vi "ProdaNG.File.Read.vi"(6 "Config":T1={"ShowUnreleased"=FALSE, "Param1"="", "ParamStartIdx"=0, "Slots"=1} {"Slots" min=1 max=2; "ParamStartIdx" min=0 max=1}, 8 "error in (no error)":errorcluster, 9 "units":T2[](array[typedef]), 10 "SeqFile Path":path, 11 "SlotNo":i32) -> (0 "error out":errorcluster, 1 "#Slots":i32, 2 "Seq":T3)   [LabVIEW 2016]
uses:
  ProdaNG.File.Sequence.ctl
  ProdaNG.Tree.Fglb.Value.ctl
  ProdaNG.File.Step.ctl
  Controls/ProdaNG.UnitSimple.ctl
  ProdaNG.Configurator.Config.ctl
  <vilib>/Utility/config.llb/Read Key (String).vi
  <vilib>/Utility/config.llb/NI_LVConfig.lvlib
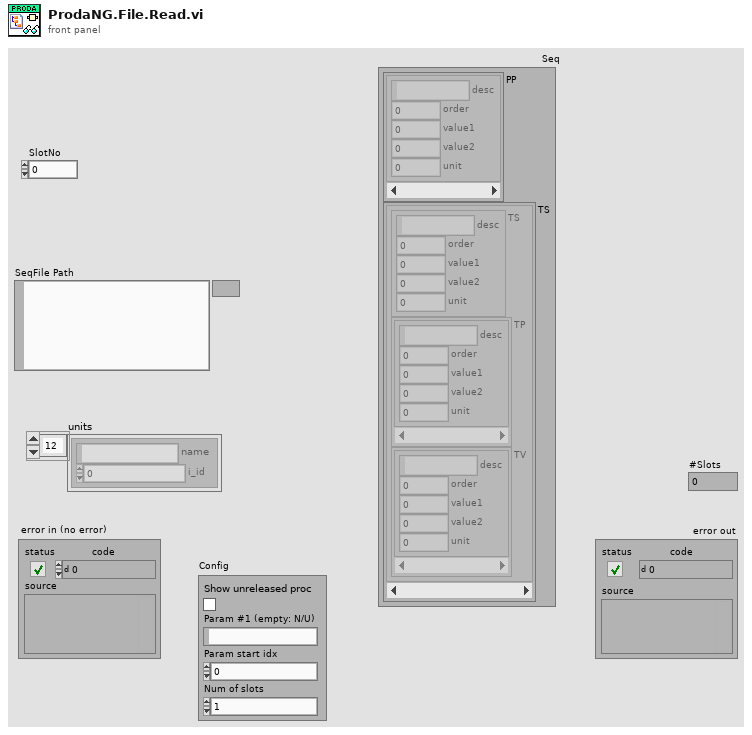
[diagram p1: front panel]
types:
  T1 = typedef "ProdaNG.Configurator.Config.ctl" = cluster{"ShowUnreleased":bool, "Param1":string, "ParamStartIdx":i32, "Slots":i32}
  T2 = typedef "ProdaNG.UnitSimple.ctl" = cluster{"name":string, "i_id":i32}
  T3 = typedef "ProdaNG.File.Sequence.ctl" = cluster{"PP":T4[], "TS":T5[]}
  T4 = typedef "ProdaNG.Tree.Fglb.Value.ctl" = cluster{"desc":string, "order":i32, "value1":dbl, "value2":dbl, "unit":i32}
  T5 = typedef "ProdaNG.File.Step.ctl" = cluster{"TS":T4, "TP":T4[], "TV":T4[]}
  T6 = typedef "NI_LVConfig.lvlib/Config Data RefNum.ctl" = refnum<k1>
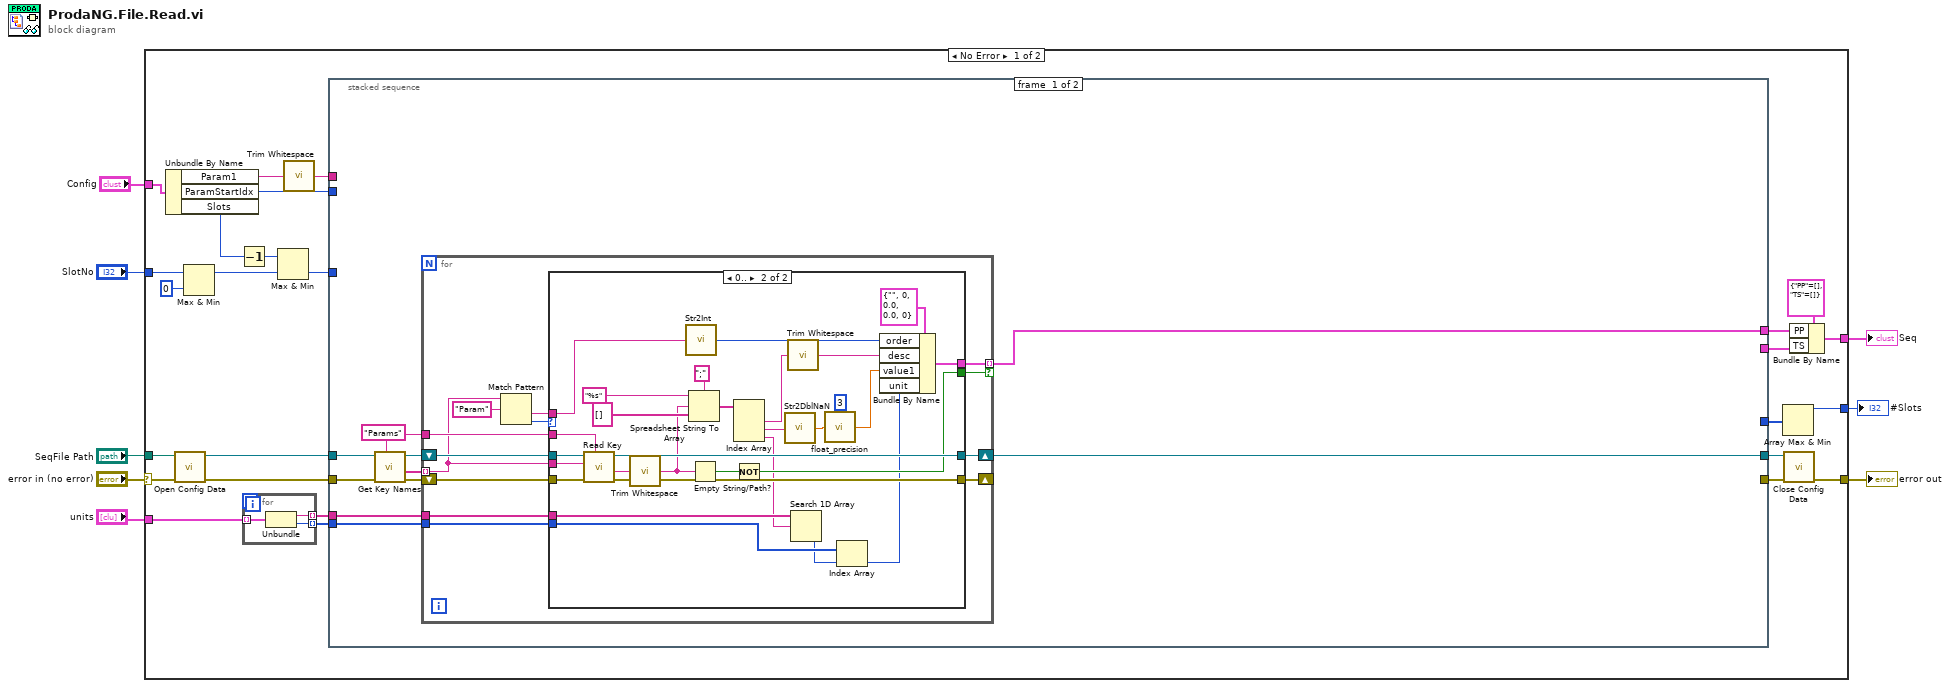
[diagram p0: block diagram]
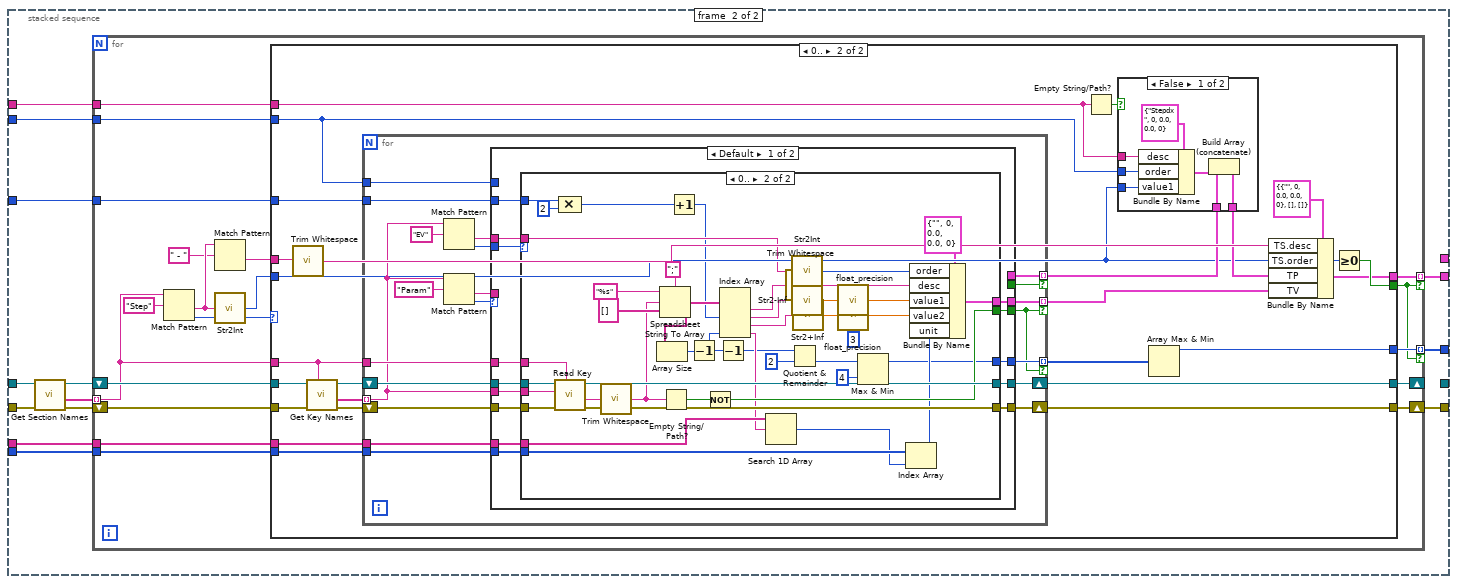
[diagram p3: hidden frame]
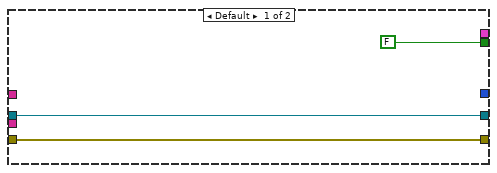
[diagram p6: hidden frame]
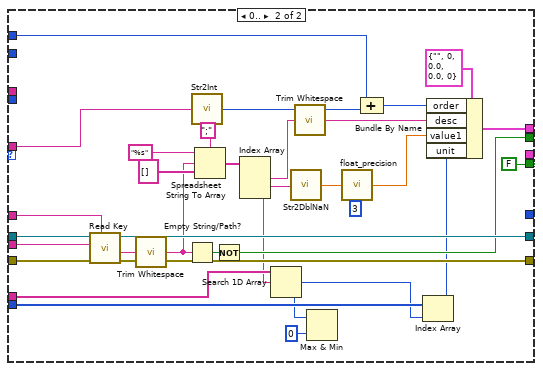
[diagram p7: hidden frame]
diagram:
  n1 = case shown="No Error" "error in (no error)" {
    selector: "error in (no error)" -> [w34 w273]
    tunnel: [w33 w273] -> w7
    tunnel: [w20 _] -> w6
    tunnel: "SeqFile Path" -> [w32 _]
    tunnel: "units" -> [w29 _]
    tunnel: "SlotNo" -> [w26 _]
    tunnel: [w18 _] -> w2
    tunnel: "Config" -> [w15 _]
    frame No Error {
      n2 = Unbundle By Name(w15) -> ("Param1"=w16:string, "ParamStartIdx"=w13:i32, "Slots"=w12:i32)
      n3 = call <vilib>:"Open Config Data.vi"("error in (no error)"=w34, "configuration file path"=w32) -> ("error out"=w31:errorcluster, "refnum"=w30:T6)  [unwired: 7 in, 1 out]
      n4 = Max & Min(x=w26, y=0) -> (max(x,y)=w10:i32)  [unwired: 1 out]
      n5 = Decrement(x=w12) -> (x-1=w11:i32)
      n6 = for {
        tunnel: [w272] -> w28 mode=indexing
        tunnel: [w271] -> w27 mode=indexing
        tunnel: w29 -> [w270] mode=indexing
        n7 = Unbundle(w270) -> ("name"=w272:string, "i_id"=w271:i32)
      }
      n8 = Max & Min(x=w11, y=w10) -> (min(x,y)=w9:i32)  [unwired: 1 out]
      n9 = call <vilib>:"Trim Whitespace.vi"("string"=w16) -> ("trimmed string"=w14:string)  [unwired: 1 in]
      n10 = stacked-sequence {
        tunnel: w31 -> [w40 w99]
        tunnel: w30 -> [w39 w98]
        tunnel: w28 -> [w38 w96]
        tunnel: w27 -> [w37 w95]
        tunnel: w9 -> [_ w94]
        tunnel: [_ w93] -> w25
        tunnel: [w36 _] -> w24
        tunnel: [_ w92] -> w22
        tunnel: [w35 _] -> w21
        tunnel: [_ w91] -> w19
        tunnel: w14 -> [_ w90]
        tunnel: w13 -> [_ w89]
        frame #0 {
          w41 = "Params" ("regular expression")
          n11 = call <vilib>:"Get Key Names.vi"("section"=w41, "error in (no error)"=w40, "refnum"=w39) -> ("error out"=w42:errorcluster, "key names"=w44:string[], "refnum out"=w43:T6)  [unwired: 5 in, 1 out]
          n12 = for {
            tunnel: w44 -> [w47] mode=indexing
            shift-right: [w50] -> w36
            shift-left: w43 -> [w54]
            shift-right: [w49] -> _
            shift-left: w42 -> [w55]
            tunnel: w41 -> [w53]
            tunnel: [w51] -> w35 mode=indexing if=w48
            tunnel: w38 -> [w46]
            tunnel: w37 -> [w45]
            n13 = Match Pattern(string=w47, regular expression="Param") -> (after substring=w52:string, offset past match=w56:i32)  [unwired: 1 in, 2 out]
            n14 = case shown="0.." w56 {
              tunnel: w55 -> [w58 w88]
              tunnel: w54 -> [w59 w87]
              tunnel: w53 -> [_ w86]
              tunnel: w47 -> [_ w85]
              tunnel: w52 -> [_ w79]
              tunnel: [_ w76] -> w51
              tunnel: [w59 w75] -> w50
              tunnel: [w58 w74] -> w49
              tunnel: [_ w71] -> w48
              tunnel: w46 -> [_ w69]
              tunnel: w45 -> [_ w67]
              frame Default {
              }
              frame 0.. {
                n15 = call-poly <vilib>:"Read Key.vi"("section"=w86, "error in (no error)"=w88, "key"=w85, "refnum"=w87) -> ("error out"=w74:errorcluster, "value"=w84:string, "refnum out"=w75:T6)  [unwired: 4 in, 1 out]
                n16 = call <vilib>:"Trim Whitespace.vi"("string"=w84) -> ("trimmed string"=w73:string)  [unwired: 1 in]
                n17 = call "Str2Int.vi"("string"=w79) -> ("Numeric"=w60:i32)
                n18 = Spreadsheet String To Array(delimiter (Tab)=";", format string="%s", spreadsheet string=w73, array type (2D Dbl)=string[] []) -> (array=w80:string[])
                n19 = Empty String/Path?(string/path=w73) -> (empty?=w72:bool)
                n20 = Index Array(array=w80) -> (element #1=w78:string, element #2=w77:string, element #3=w68:string)  [unwired: 3 in]
                n21 = Not(x=w72) -> (.not. x?=w71:bool)
                n22 = call "Str2DblNaN.vi"("string"=w77) -> ("Numeric"=w64:dbl)
                n23 = call <vilib>:"Trim Whitespace.vi"("string"=w78) -> ("trimmed string"=w65:string)  [unwired: 1 in]
                n24 = Search 1D Array(1D array=w69, element=w68) -> (index of element=w66:i32)  [unwired: 1 in]
                n25 = call "float_precision.vi"("input"=w64, "precision"=3) -> ("output"=w63:dbl)
                n26 = Index Array(array=w67, index=w66) -> (element=w61:i32)
                n27 = Bundle By Name(cluster=T4 {"desc"="", "order"=0, "value1"=0.0, "value2"=0.0, "unit"=0} ("Element values"), "order"=w60, "desc"=w65, "value1"=w63, "unit"=w61) -> (w76:T4)
              }
            }
          }
        }
        frame #1 {
          n28 = call <vilib>:"Get Section Names.vi"("error in (no error)"=w99, "refnum"=w98) -> ("error out"=w100:errorcluster, "section names"=w101:string[], "refnum out"=w97:T6)  [unwired: 7 in]
          n29 = for {
            tunnel: w101 -> [w114] mode=indexing
            shift-right: [w117] -> w93
            shift-left: w100 -> [w118]
            shift-right: [w115] -> _
            shift-left: w97 -> [w116]
            tunnel: [w113] -> w92 mode=indexing if=w104
            tunnel: w96 -> [w108]
            tunnel: w95 -> [w107]
            tunnel: w94 -> [w106]
            tunnel: [w105] -> w91 mode=indexing if=w104
            tunnel: w90 -> [w103]
            tunnel: w89 -> [w102]
            n30 = Match Pattern(string=w114, regular expression="Step") -> (after substring=w111:string, offset past match=w119:i32)  [unwired: 1 in, 2 out]
            n31 = Match Pattern(string=w111, regular expression=" - ") -> (after substring=w109:string)  [unwired: 1 in, 3 out]
            n32 = call "Str2Int.vi"("string"=w111) -> ("Numeric"=w112:i32)
            n33 = case shown="0.." w119 {
              tunnel: [w122 w139] -> w117
              tunnel: w118 -> [w122 w146]
              tunnel: w116 -> [w121 w147]
              tunnel: [w121 w140] -> w115
              tunnel: w114 -> [_ w142]
              tunnel: [_ w136] -> w113
              tunnel: w112 -> [_ w128]
              tunnel: [_ w138] -> w104
              tunnel: w109 -> [_ w137]
              tunnel: w108 -> [_ w134]
              tunnel: w107 -> [_ w133]
              tunnel: w106 -> [_ w132]
              tunnel: [_ w126] -> w105
              tunnel: w103 -> [_ w124]
              tunnel: w102 -> [_ w123]
              frame Default {
              }
              frame 0.. {
                n34 = call <vilib>:"Trim Whitespace.vi"("string"=w137) -> ("trimmed string"=w135:string)  [unwired: 1 in]
                n35 = call <vilib>:"Get Key Names.vi"("section"=w142, "error in (no error)"=w146, "refnum"=w147) -> ("error out"=w143:errorcluster, "key names"=w145:string[], "refnum out"=w144:T6)  [unwired: 5 in, 1 out]
                n36 = for {
                  tunnel: w145 -> [w164] mode=indexing
                  shift-right: [w169] -> w140
                  shift-left: w144 -> [w173]
                  shift-right: [w168] -> w139
                  shift-left: w143 -> [w174]
                  tunnel: w142 -> [w172]
                  tunnel: [w170] -> w130 mode=indexing if=w167
                  tunnel: [w166] -> w141 mode=indexing if=w157
                  tunnel: w134 -> [w161]
                  tunnel: w133 -> [w160]
                  tunnel: w132 -> [w159]
                  tunnel: [w158] -> w127 mode=indexing if=w157
                  tunnel: w123 -> [w156]
                  n37 = Match Pattern(string=w164, regular expression="EV") -> (after substring=w162:string, offset past match=w163:i32)  [unwired: 1 in, 2 out]
                  n38 = Match Pattern(string=w164, regular expression="Param") -> (after substring=w171:string, offset past match=w175:i32)  [unwired: 1 in, 2 out]
                  n39 = case shown="Default" w175 {
                    tunnel: w174 -> [w190 w269]
                    tunnel: w173 -> [w189 w268]
                    tunnel: w172 -> [w184 w267]
                    tunnel: w164 -> [w183 w266]
                    tunnel: w171 -> [_ w260]
                    tunnel: [_ w257] -> w170
                    tunnel: [w188 w256] -> w169
                    tunnel: [w187 w255] -> w168
                    tunnel: [_ w252] -> w167
                    tunnel: [w186 _] -> w166
                    tunnel: [w185 FALSE] -> w157
                    tunnel: w163 -> [w182 _]
                    tunnel: w162 -> [w181 _]
                    tunnel: w161 -> [w180 w249]
                    tunnel: w160 -> [w179 w247]
                    tunnel: w159 -> [w178 _]
                    tunnel: [w177 _] -> w158
                    tunnel: w156 -> [_ w237]
                    frame Default {
                      n40 = case shown="0.." w182 {
                        tunnel: w190 -> [w192 w236]
                        tunnel: w189 -> [w193 w235]
                        tunnel: w184 -> [_ w234]
                        tunnel: w183 -> [_ w233]
                        tunnel: w181 -> [_ w211]
                        tunnel: [_ w226] -> w186
                        tunnel: [w193 w225] -> w188
                        tunnel: [w192 w224] -> w187
                        tunnel: [FALSE w221] -> w185
                        tunnel: w180 -> [_ w220]
                        tunnel: w179 -> [_ w219]
                        tunnel: w178 -> [_ w202]
                        tunnel: [_ w195] -> w177
                        frame Default {
                        }
                        frame 0.. {
                          w205 = 3 ("precision")
                          n41 = call-poly <vilib>:"Read Key.vi"("section"=w234, "error in (no error)"=w236, "key"=w233, "refnum"=w235) -> ("error out"=w224:errorcluster, "value"=w232:string, "refnum out"=w225:T6)  [unwired: 4 in, 1 out]
                          n42 = Compound Arithmetic op=MULTIPLY(w202, 2 ("value")) -> (w200:i32)
                          n43 = call <vilib>:"Trim Whitespace.vi"("string"=w232) -> ("trimmed string"=w223:string)  [unwired: 1 in]
                          n44 = Spreadsheet String To Array(delimiter (Tab)=";", format string="%s", spreadsheet string=w223, array type (2D Dbl)=string[] []) -> (array=w217:string[])
                          n45 = Array Size(array=w217) -> (size(s)=w214:i32)
                          n46 = Empty String/Path?(string/path=w223) -> (empty?=w222:bool)
                          n47 = Increment(x=w200) -> (x+1=w199:i32)
                          n48 = Decrement(x=w214) -> (x-1=w203:i32)
                          n49 = Not(x=w222) -> (.not. x?=w221:bool)
                          n50 = Decrement(x=w203) -> (x-1=w198:i32)
                          n51 = Index Array(array=w217, index #2=w199, index #4=w203) -> (element #1=w227:string, element #2=w215:string, element #3=w216:string, element #4=w213:string)  [unwired: 2 in]
                          n52 = Search 1D Array(1D array=w220, element=w213) -> (index of element=w204:i32)  [unwired: 1 in]
                          n53 = call <vilib>:"Trim Whitespace.vi"("string"=w227) -> ("trimmed string"=w210:string)  [unwired: 1 in]
                          n54 = Quotient & Remainder(x=w198, y=2) -> (floor(x/y)=w196:i32)  [unwired: 1 out]
                          n55 = call "Str2Int.vi"("string"=w211) -> ("Numeric"=w228:i32)
                          n56 = call "Str2-Inf.vi"("string"=w215) -> ("Numeric"=w209:dbl)
                          n57 = call "Str2+Inf.vi"("string"=w216) -> ("Numeric"=w207:dbl)
                          n58 = call "float_precision.vi"("input"=w209, "precision"=w205) -> ("output"=w208:dbl)
                          n59 = call "float_precision.vi"("input"=w207, "precision"=w205) -> ("output"=w206:dbl)
                          n60 = Max & Min(x=w196, y=4) -> (max(x,y)=w195:i32)  [unwired: 1 out]
                          n61 = Index Array(array=w219, index=w204) -> (element=w212:i32)
                          n62 = Bundle By Name(cluster=T4 {"desc"="", "order"=0, "value1"=0.0, "value2"=0.0, "unit"=0} ("Element values"), "order"=w228, "desc"=w210, "value1"=w208, "value2"=w206, "unit"=w212) -> (w226:T4)
                        }
                      }
                    }
                    frame 0.. {
                      n63 = call-poly <vilib>:"Read Key.vi"("section"=w267, "error in (no error)"=w269, "key"=w266, "refnum"=w268) -> ("error out"=w255:errorcluster, "value"=w265:string, "refnum out"=w256:T6)  [unwired: 4 in, 1 out]
                      n64 = call <vilib>:"Trim Whitespace.vi"("string"=w265) -> ("trimmed string"=w254:string)  [unwired: 1 in]
                      n65 = Empty String/Path?(string/path=w254) -> (empty?=w253:bool)
                      n66 = call "Str2Int.vi"("string"=w260) -> ("Numeric"=w240:i32)
                      n67 = Spreadsheet String To Array(delimiter (Tab)=";", format string="%s", spreadsheet string=w254, array type (2D Dbl)=string[] []) -> (array=w261:string[])
                      n68 = Not(x=w253) -> (.not. x?=w252:bool)
                      n69 = Index Array(array=w261) -> (element #1=w259:string, element #2=w258:string, element #3=w248:string)  [unwired: 3 in]
                      n70 = Search 1D Array(1D array=w249, element=w248) -> (index of element=w239:i32)  [unwired: 1 in]
                      n71 = call "Str2DblNaN.vi"("string"=w258) -> ("Numeric"=w243:dbl)
                      n72 = call <vilib>:"Trim Whitespace.vi"("string"=w259) -> ("trimmed string"=w245:string)  [unwired: 1 in]
                      n73 = Max & Min(x=w239, y=0) -> ()  [unwired: 2 out]
                      n74 = call "float_precision.vi"("input"=w243, "precision"=3) -> ("output"=w242:dbl)
                      n75 = Compound Arithmetic op=ADD(w237, w240) -> (w238:i32)
                      n76 = Index Array(array=w247, index=w239) -> (element=w246:i32)
                      n77 = Bundle By Name(cluster=T4 {"desc"="", "order"=0, "value1"=0.0, "value2"=0.0, "unit"=0} ("Element values"), "order"=w238, "desc"=w245, "value1"=w242, "unit"=w246) -> (w257:T4)
                    }
                  }
                }
                n78 = Empty String/Path?(string/path=w124) -> (empty?=w125:bool)
                n79 = case shown="False" w125 {
                  tunnel: w130 -> [w153 w155]
                  tunnel: [w152 w155] -> w129
                  tunnel: w128 -> [w151 _]
                  tunnel: w124 -> [w149 _]
                  tunnel: w123 -> [w148 _]
                  frame False {
                    n80 = Bundle By Name(cluster=T4 {"desc"="Stepdx", "order"=0, "value1"=0.0, "value2"=0.0, "unit"=0} ("Element values"), "desc"=w149, "order"=w148, "value1"=w151) -> (w154:T4)
                    n81 = Build Array (concatenate)(w154, w153) -> (w152:T4[])
                  }
                  frame True {
                  }
                }
                n82 = Array Max & Min(array=w127) -> (max value=w126:i32)  [unwired: 3 out]
                n83 = Bundle By Name(cluster=T5 {"TS"={"desc"="", "order"=0, "value1"=0.0, "value2"=0.0, "unit"=0}, "TP"=[], "TV"=[]} ("Step"), "TS.desc"=w135, "TS.order"=w128, "TP"=w129, "TV"=w141) -> (w136:T5)
                n84 = Greater Or Equal To 0?(x=w128) -> (x >= 0?=w138:bool)
              }
            }
          }
        }
      }
      n85 = Array Max & Min(array=w19) -> (max value=w18:i32)  [unwired: 3 out]
      n86 = call <vilib>:"Close Config Data.vi"("error in (no error)"=w25, "refnum"=w24) -> ("error out"=w33:errorcluster)  [unwired: 8 in, 1 out]
      n87 = Bundle By Name(cluster=T3 {"PP"=[], "TS"=[]} ("Seq"), "PP"=w21, "TS"=w22) -> (w20:T3)
    }
    frame Error {
    }
  }
  "error out" <- w7
  "Seq" <- w6
  "#Slots" <- w2
